vi "SubVI_Filter_EEG_Debug.vi"(4 "EEG":T1, 8 "error in (no error)":errorcluster, 9 "Resampling rate":dbl, 10 "Interpolant Size":dbl) -> (0 "error out":errorcluster, 3 "Filtered EEG Out":T2)   [LabVIEW 2020]
uses:
  <extravilib>/ChannelInstances/Stream-a[.,.](dbl)/)Channel.ctl
  <extravilib>/ChannelInstances/Stream-a[.](dbl)/)Channel.ctl
  <vilib>/Analysis/3filter.llb/Filter Passband Type.ctl
  <extravilib>/ChannelInstances/Stream-a[.](dbl)/EndpointRead.vi
  <extravilib>/ChannelInstances/Stream-a[.,.](dbl)/Endpoint.vi
  Global 1.vi
  <extravilib>/ChannelInstances/Stream-a[.](dbl)/)Channel.vi
  <resource>/ChannelSupport/_ChannelSupport/WaitIfNeeded.vi
  <extravilib>/ChannelInstances/Stream-a[.,.](dbl)/)Channel.vi
  <vilib>/Analysis/NI_AALBase.lvlib
  <vilib>/ptbypt/NI_PtbyPt.lvlib
  <extravilib>/ChannelInstances/Stream-a[.,.](dbl).lvlib
  <extravilib>/ChannelInstances/Stream-a[.](dbl).lvlib
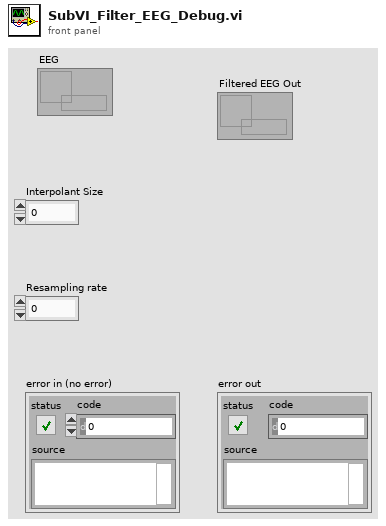
[diagram p1: front panel]
types:
  T1 = typedef "Stream-a[.](dbl).lvlib/)Channel.ctl" = refnum<queue>
  T2 = typedef "Stream-a[.,.](dbl).lvlib/)Channel.ctl" = refnum<queue>
  T3 = typedef "NI_AALBase.lvlib/Filter Passband Type.ctl" = enum32{"Lowpass", "Highpass", "Bandpass", "Bandstop"}
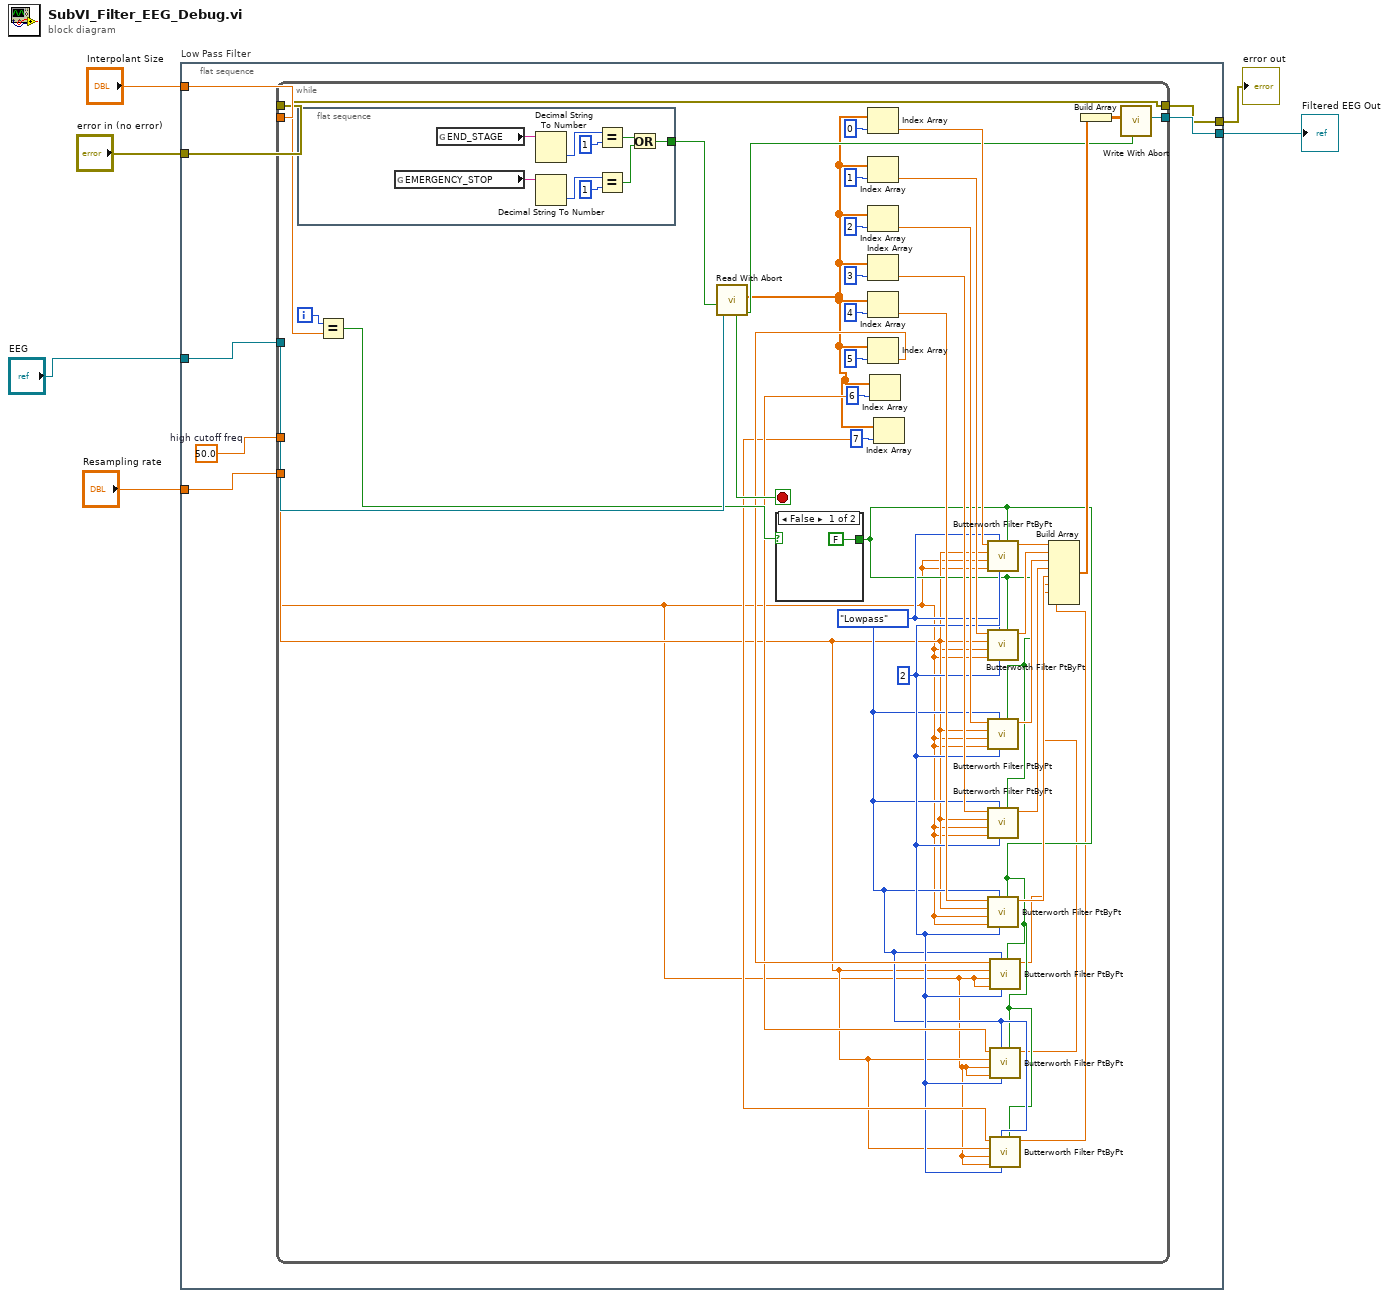
[diagram p0: block diagram]
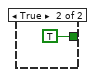
[diagram p2: hidden frame]
diagram:
  n1 = flat-sequence "Low Pass Filter" {
    tunnel: "EEG" -> [w13]
    tunnel: [w12] -> w4
    tunnel: "Interpolant Size" -> [w11]
    tunnel: "Resampling rate" -> [w10]
    tunnel: "error in (no error)" -> [w8]
    tunnel: [w7] -> w2
    frame #0 {
      w9 = 50.0  # high cutoff freq
      n2 = while {
        tunnel: w13 -> [w39]
        tunnel: [w38] -> w12
        tunnel: w11 -> [w36]
        tunnel: w9 -> [w18]
        tunnel: w10 -> [w19]
        tunnel: w8 -> [w29]
        tunnel: [w29] -> w7
        i -> [w37]
        stop <- w31 stop-if-true
        w22 = 2 ("order")
        w21 = Filter_Passband_Type."Lowpass" ("filter type")
        n3 = flat-sequence {
          tunnel: [w54] -> w30
          frame #0 {
            n4 = global read "Global 1.vi" "EMERGENCY_STOP"() -> (w57:string)
            n5 = global read "Global 1.vi" "END_STAGE"() -> (w62:string)
            n6 = Decimal String To Number(string=w62) -> (number=w61:i32)  [unwired: 2 in, 1 out]
            n7 = Decimal String To Number(string=w57) -> (number=w59:i32)  [unwired: 2 in, 1 out]
            n8 = Equal?(x=w61, y=1) -> (x = y?=w55:bool)
            n9 = Equal?(x=w59, y=1) -> (x = y?=w56:bool)
            n10 = Or(x=w55, y=w56) -> (x .or. y?=w54:bool)
          }
        }
        n11 = Equal?(x=w37, y=w36) -> (x = y?=w35:bool)
        n12 = call <extravilib>:"Read With Abort.vi"("abort"=w30, "channel"=w39) -> ("element"=w14:dbl[], "aborted?"=w31:bool)  [unwired: 4 in, 4 out]
        n13 = case shown="False" w35 {
          tunnel: [FALSE ("init/cont (init:F)") TRUE ("init/cont (init:F)")] -> w20
          frame False {
          }
          frame True {
          }
        }
        n14 = Index Array(array=w14, index=0 ("disabled index (col)")) -> (element=w48:dbl)
        n15 = Index Array(array=w14, index=1 ("disabled index (col)")) -> (element=w49:dbl)
        n16 = Index Array(array=w14, index=2 ("disabled index (col)")) -> (element=w50:dbl)
        n17 = Index Array(array=w14, index=3 ("disabled index (col)")) -> (element=w51:dbl)
        n18 = Index Array(array=w14, index=4 ("disabled index (col)")) -> (element=w34:dbl)
        n19 = Index Array(array=w14, index=5 ("disabled index (col)")) -> (element=w25:dbl)
        n20 = Index Array(array=w14, index=6 ("disabled index (col)")) -> (element=w24:dbl)
        n21 = Index Array(array=w14, index=7 ("disabled index (col)")) -> (element=w23:dbl)
        n22 = call <vilib>:"Butterworth Filter PtByPt.vi"("initialize"=w20, "order"=w22, "filter type"=w21, "low cutoff freq: fl"=w18, "high cutoff freq: fh"=w18, "sampling freq: fs"=w19, "x"=w48) -> ("Filtered x"=w44:dbl)  [unwired: 2 in, 1 out]
        n23 = call <vilib>:"Butterworth Filter PtByPt.vi"("initialize"=w20, "order"=w22, "filter type"=w21, "low cutoff freq: fl"=w18, "high cutoff freq: fh"=w18, "sampling freq: fs"=w19, "x"=w49) -> ("Filtered x"=w45:dbl)  [unwired: 2 in, 1 out]
        n24 = call <vilib>:"Butterworth Filter PtByPt.vi"("initialize"=w20, "order"=w22, "filter type"=w21, "low cutoff freq: fl"=w18, "high cutoff freq: fh"=w18, "sampling freq: fs"=w19, "x"=w50) -> ("Filtered x"=w46:dbl)  [unwired: 2 in, 1 out]
        n25 = call <vilib>:"Butterworth Filter PtByPt.vi"("initialize"=w20, "order"=w22, "filter type"=w21, "low cutoff freq: fl"=w18, "high cutoff freq: fh"=w18, "sampling freq: fs"=w19, "x"=w51) -> ("Filtered x"=w47:dbl)  [unwired: 2 in, 1 out]
        n26 = call <vilib>:"Butterworth Filter PtByPt.vi"("initialize"=w20, "order"=w22, "filter type"=w21, "low cutoff freq: fl"=w18, "high cutoff freq: fh"=w18, "sampling freq: fs"=w19, "x"=w34) -> ("Filtered x"=w32:dbl)  [unwired: 2 in, 1 out]
        n27 = call <vilib>:"Butterworth Filter PtByPt.vi"("initialize"=w20, "order"=w22, "filter type"=w21, "low cutoff freq: fl"=w18, "high cutoff freq: fh"=w18, "sampling freq: fs"=w19, "x"=w25) -> ("Filtered x"=w17:dbl)  [unwired: 2 in, 1 out]
        n28 = call <vilib>:"Butterworth Filter PtByPt.vi"("initialize"=w20, "order"=w22, "filter type"=w21, "low cutoff freq: fl"=w18, "high cutoff freq: fh"=w18, "sampling freq: fs"=w19, "x"=w24) -> ("Filtered x"=w16:dbl)  [unwired: 2 in, 1 out]
        n29 = call <vilib>:"Butterworth Filter PtByPt.vi"("initialize"=w20, "order"=w22, "filter type"=w21, "low cutoff freq: fl"=w18, "high cutoff freq: fh"=w18, "sampling freq: fs"=w19, "x"=w23) -> ("Filtered x"=w15:dbl)  [unwired: 2 in, 1 out]
        n30 = Build Array(w44, w45, w46, w47, w32, w17, w16, w15) -> (w52:dbl[])
        n31 = Build Array(w52) -> (w53:dbl[][])
        n32 = call <extravilib>:"Write With Abort.vi"("abort"=w31, "element"=w53) -> ("channel"=w38:T2)  [unwired: 6 in, 3 out]
      }
    }
  }
  "Filtered EEG Out" <- w4
  "error out" <- w2
